vi "Release.vi"(8 "error in (no error)":errorcluster, 11 "Mapped Memory Access Image ARGB":refnum<data-value>) -> (0 "error out":errorcluster, 3 "Image ARGB":refnum<data-value>)   [LabVIEW 2020, in "g_ar_toolkit.image.lvlib" / "Mapped Memory Access Image ARGB.lvclass"]
uses:
  Mapped Memory Access Image ARGB.lvclass
  Mapped Memory Access Image ARGB.lvclass/Mapped Memory Access Image ARGB.ctl
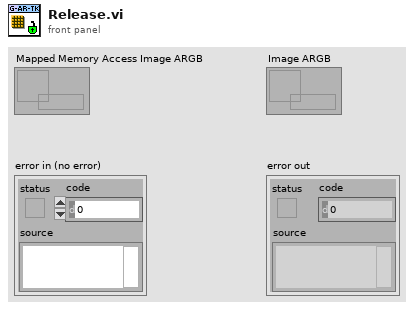
[diagram p1: front panel]
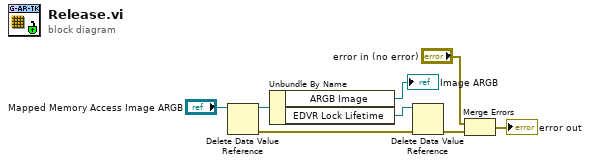
[diagram p0: block diagram]
diagram:
  n1 = Delete Data Value Reference(data value reference="Mapped Memory Access Image ARGB") -> (data value=w6:refnum<class "Mapped Memory Access Image ARGB.lvclass">, error out=w2:errorcluster)  [unwired: 1 in]
  n2 = Unbundle By Name(w6) -> ("ARGB Image"=→"Image ARGB":refnum<data-value>, "EDVR Lock Lifetime"=w3:refnum<data-value>)
  n3 = Delete Data Value Reference(data value reference=w3, error in=w2) -> (error out=w1:errorcluster)  [unwired: 1 out]
  n4 = Merge Errors("error in (no error)", w1) -> (→"error out":errorcluster)
